vi "Write Pulse Controller Configuration.vi"(8 "error in (no error)":errorcluster, 10 "Configuration":T1={"Pre-trigger duration"=-1.0, "Post-trigger duration"=-1.0, "Open plot after pulse"=FALSE} {"Pre-trigger duration" format="%#_6p"; "Post-trigger duration" format="%#_6p"}, 11 "Pulse Controller in":refnum<class "Pulse Controller.lvclass">) -> (0 "error out":errorcluster, 3 "Pulse Controller out":refnum<class "Pulse Controller.lvclass">)   [LabVIEW 2015, in "Pulse Controller.lvclass"]
uses:
  Pulse Controller.lvclass
  Pulse Controller Configuration.ctl
  Measure Object/Measure Object.lvclass/Measure Object.ctl
  Measure Object/Write Configuration.vi
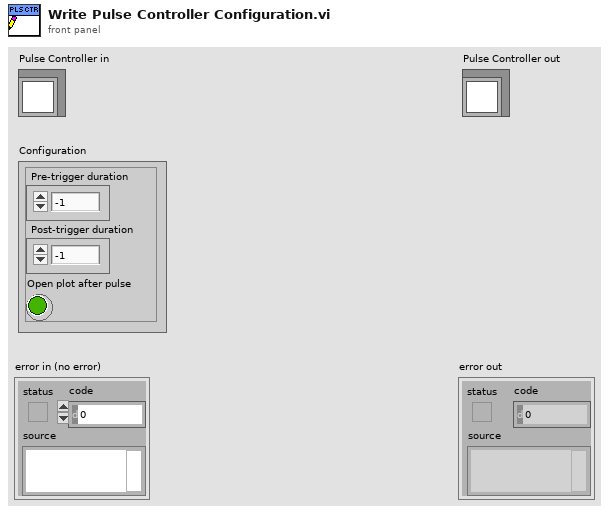
[diagram p1: front panel]
types:
  T1 = typedef "Pulse Controller Configuration.ctl" = cluster{"Pre-trigger duration":dbl, "Post-trigger duration":dbl, "Open plot after pulse":bool}
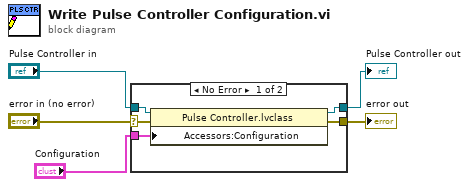
[diagram p0: block diagram]
diagram:
  n1 = case shown="No Error" "error in (no error)" {
    selector: "error in (no error)" -> [w7 w11]
    tunnel: [w6 w11] -> w4
    tunnel: [w9 w12] -> w2
    tunnel: "Pulse Controller in" -> [w10 w12]
    tunnel: "Configuration" -> [w8 _]
    frame No Error {
      n2 = property class="Pulse Controller.lvclass"(reference=w10, error in=w7, "Accessors:Configuration"=w8) -> (reference out=w9:refnum<class "Pulse Controller.lvclass">, error out=w6:errorcluster)
    }
    frame Error {
    }
  }
  "error out" <- w4
  "Pulse Controller out" <- w2
